vi "send lab ambient data to processor.vi"(8 "error in (no error)":errorcluster, 10 "RT Queues":T1, 11 "read data":T2) -> ()   [LabVIEW 2018]
uses:
  ICL-LabVIEW_General/Main Controller SVE/SharedResourceCtrls/MainCabinetDataRead.ctl
  Type Defs/Queues cluster.ctl
  ICL-LabVIEW_General/Message Scheduler/message scheduler.lvclass
  Queue VIs/En-queue RT data element.vi
  ICL-LabVIEW_General/Main Controller SVE/Lab123H main cabinet API.lvlib
panel:
  out "Lab Temperature":dbl
  out "Lab Pressure":sgl
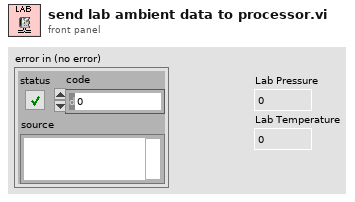
[diagram p1: front panel]
types:
  T1 = typedef "Queues cluster.ctl" = cluster{"RT Message":refnum<queue>, "RT Comms":refnum<queue>, "RT Data":refnum<queue>, "RT FIFO":refnum<queue>, "message scheduler":refnum<class "message scheduler.lvclass">}
  T2 = typedef "Lab123H main cabinet API.lvlib/MainCabinetDataRead.ctl" = cluster{"CurrentIn":cluster{"MainValveFeed(%)":sgl, "SecValveFeed(%)":sgl, "AirMassFlow(Kg/s)":sgl, "StatorOilPressure(BarG)":sgl, "BearingOilPressure(BarG)":sgl}, "VoltageIn":cluster{"AmbientPressure(Pa)":sgl}, "Indicators":cluster{"AirMassFlowOK":bool, "EMstopOK":bool, "Thermocouple Error":bool, "MainCabinet_CPU (%)":dbl, "Error":bool}, "Temperature":cluster{"LabTemp":dbl, "HeaterTemp":dbl, "Oil TC 1":dbl, "Oil TC 2":dbl, "Oil TC 3":dbl, "Oil TC 4":dbl, "Oil TC 5":dbl, "Oil TC 6":dbl}, "Flowrates (L/min)":cluster{"BearingOil":dbl, "StatorOil":dbl, "BearingFlow":bool, "StatorFlow":bool}}
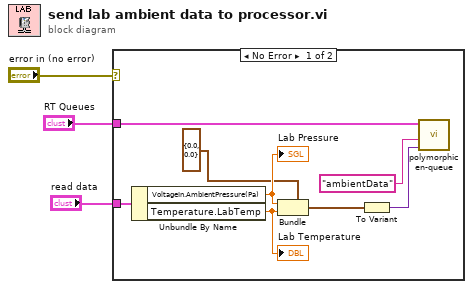
[diagram p0: block diagram]
diagram:
  n1 = case shown="No Error" "error in (no error)" {
    tunnel: "RT Queues" -> [w11 _]
    tunnel: "read data" -> [w10 _]
    frame No Error {
      n2 = Unbundle By Name(w10) -> ("VoltageIn.AmbientPressure(Pa)"=w9:sgl, "Temperature.LabTemp"=w8:dbl)
      "Lab Pressure" <- w9
      "Lab Temperature" <- w8
      n3 = Bundle(cluster=cluster{"pressure":dbl, "temperature":dbl} {"pressure"=0.0, "temperature"=0.0} ("labAmbient"), "pressure"=w9, "temperature"=w8) -> (w4:cluster{"pressure":dbl, "temperature":dbl})
      n4 = To Variant(anything=w4) -> (Variant=w7:variant)
      n5 = call-poly "polymorphic en-queue.vi"("Data"=w7, "Message"="ambientData", "RT Queues"=w11) -> ()  [unwired: 6 in, 3 out]
    }
    frame Error {
    }
  }
